vi "WalkOnTests.vi"(6 "Stop on 1st fail":bool, 7 "Banana":refnum<class "Banana.lvclass">, 8 "error in (no error)":errorcluster, 10 "Properties.Test":refnum<class "Properties.Test.lvclass">) -> (0 "error out":errorcluster, 2 "Properties.Test out":refnum<class "Properties.Test.lvclass">)   [LabVIEW 2021, in "Bananas.lvlib" / "Platano.lvclass"]
uses:
  Platano.lvclass
  <vilib>/addons/_JKI Toolkits/Caraya/classes/Properties.Test/Properties.Test.lvclass
  Banana/Banana.lvclass
  Banana/Banana.lvclass/Banana.ctl
  BananaPeel/BananaPeel.lvclass
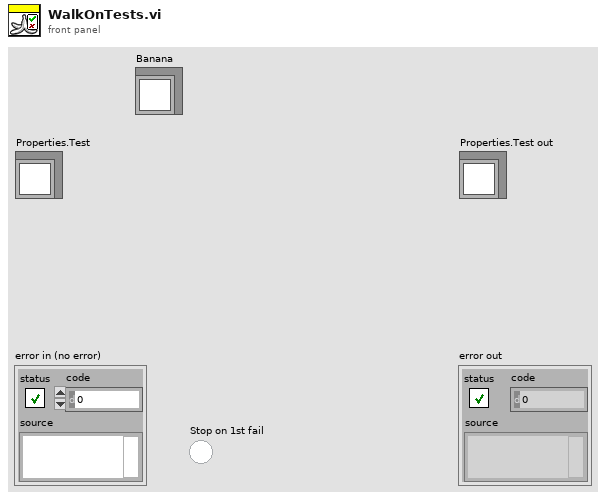
[diagram p1: front panel]
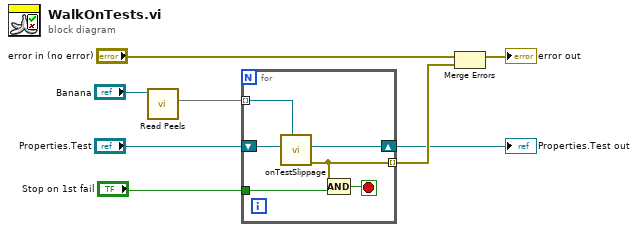
[diagram p0: block diagram]
diagram:
  n1 = call "Read Peels.vi"("Banana in"="Banana") -> ("Peels"=w1:set{refnum<class "BananaPeel.lvclass">})  [unwired: 8 in, 2 out]
  n2 = for {
    tunnel: [w11] -> w8 mode=indexing
    shift-right: [w12] -> w5
    shift-left: "Properties.Test" -> [w13]
    tunnel: w1 -> [w14] mode=indexing
    tunnel: "Stop on 1st fail" -> [w10]
    stop <- w9 stop-if-true
    n3 = call-dynamic "onTestSlippage.vi"("BananaPeel in"=w14, "Properties.Test"=w13) -> ("error out"=w11:errorcluster, "Properties.Test out"=w12:refnum<class "Properties.Test.lvclass">)  [unwired: 8 in]
    n4 = Compound Arithmetic op=AND(w11, w10) -> (w9:bool)
  }
  "Properties.Test out" <- w5
  n5 = Merge Errors("error in (no error)", w8) -> (→"error out":errorcluster)
